vi "CRYSelect Signal Type Dialog.vi"(6 "Channel Info In":T1[](array[typedef]) {"Coupling" items=["Default"=-1, "RSE"=10083, "NRSE"=10078, "Differential"=10106, "Pseudodifferential"=12529]; "term config" items=["Default"=-1, "RSE"=10083, "NRSE"=10078, "Differential"=10106, "Pseudodifferential"=12529]; "Anti-aliasing Factor (%fs)" format="%.2f"}, 8 "Selected Signal Type In":string[](array[string]), 9 "Mode(0ne or More)":bool, 10 "I/O Calibration In":T5 {"Calibration 2D"."Sens Curve"."Z data" items=["dB", "Lin"]; "Calibration 2D"."Sens Curve"."X data" items=["dB", "Lin"]; "Calibration 2D"."Sens Curve"."Y data" items=["dB", "Lin"]; "Calibration 2D"."Sens Curve"."Z dB ref" format="%.1f"; "Calibration 2D"."Sens Curve"."Z axis" items=["Log", "Lin"]; "Calibration 2D"."Sens Curve"."X dB ref" format="%.1f"; "Calibration 2D"."Sens Curve"."X axis" items=["Log", "Lin"]; "Calibration 2D"."Sens Curve"."Y axis" items=["Log", "Lin"]; "Calibration 2D"."Sens Curve"."Y dB ref" format="%.1f"; "Calibration 2D"."Sens Curve"."Curve"."z" format="%.2f"; "Calibration 2D"."Sens Curve"."Curve"."y" format="%.2f"; "Calibration 2D"."Sens Curve"."Curve"."x" format="%.2f"; "Calibration 2D"."EQ Curve"."Z data" items=["dB", "Lin"]; "Calibration 2D"."EQ Curve"."X data" items=["dB", "Lin"]; "Calibration 2D"."EQ Curve"."Y data" items=["dB", "Lin"]; "Calibration 2D"."EQ Curve"."Z dB ref" format="%.1f"; "Calibration 2D"."EQ Curve"."Z axis" items=["Log", "Lin"]; "Calibration 2D"."EQ Curve"."X dB ref" format="%.1f"; "Calibration 2D"."EQ Curve"."X axis" items=["Log", "Lin"]; "Calibration 2D"."EQ Curve"."Y axis" items=["Log", "Lin"]; "Calibration 2D"."EQ Curve"."Y dB ref" format="%.1f"; "Calibration 2D"."EQ Curve"."Curve"."z" format="%.2f"; "Calibration 2D"."EQ Curve"."Curve"."y" format="%.2f"; "Calibration 2D"."EQ Curve"."Curve"."x" format="%.2f"; "Calibration 2D"."Corr Curve"."Z data" items=["dB", "Lin"]; "Calibration 2D"."Corr Curve"."X data" items=["dB", "Lin"]; "Calibration 2D"."Corr Curve"."Y data" items=["dB", "Lin"]; "Calibration 2D"."Corr Curve"."Z dB ref" format="%.1f"; "Calibration 2D"."Corr Curve"."Z axis" items=["Log", "Lin"]; "Calibration 2D"."Corr Curve"."X dB ref" format="%.1f"; "Calibration 2D"."Corr Curve"."X axis" items=["Log", "Lin"]; "Calibration 2D"."Corr Curve"."Y axis" items=["Log", "Lin"]; "Calibration 2D"."Corr Curve"."Y dB ref" format="%.1f"; "Calibration 2D"."Corr Curve"."Curve"."z" format="%.2f"; "Calibration 2D"."Corr Curve"."Curve"."y" format="%.2f"; "Calibration 2D"."Corr Curve"."Curve"."x" format="%.2f"; "Calibration 2D"."Calibration"."EQ Step size" items=["R10", "R20", "R40", "R80", "User"]; "Calibration 2D"."Calibration"."Corr Step size" items=["R10", "R20", "R40", "R80", "User"]}, 11 "In/Out Signal Type":bool) -> (1 "Calibration 2D Out":T2[](array[typedef]) {"Sens Curve"."Z data" items=["dB", "Lin"]; "Sens Curve"."X data" items=["dB", "Lin"]; "Sens Curve"."Y data" items=["dB", "Lin"]; "Sens Curve"."Z dB ref" format="%.1f"; "Sens Curve"."Z axis" items=["Log", "Lin"]; "Sens Curve"."X dB ref" format="%.1f"; "Sens Curve"."X axis" items=["Log", "Lin"]; "Sens Curve"."Y axis" items=["Log", "Lin"]; "Sens Curve"."Y dB ref" format="%.1f"; "Sens Curve"."Curve"."z" format="%.2f"; "Sens Curve"."Curve"."y" format="%.2f"; "Sens Curve"."Curve"."x" format="%.2f"; "EQ Curve"."Z data" items=["dB", "Lin"]; "EQ Curve"."X data" items=["dB", "Lin"]; "EQ Curve"."Y data" items=["dB", "Lin"]; "EQ Curve"."Z dB ref" format="%.1f"; "EQ Curve"."Z axis" items=["Log", "Lin"]; "EQ Curve"."X dB ref" format="%.1f"; "EQ Curve"."X axis" items=["Log", "Lin"]; "EQ Curve"."Y axis" items=["Log", "Lin"]; "EQ Curve"."Y dB ref" format="%.1f"; "EQ Curve"."Curve"."z" format="%.2f"; "EQ Curve"."Curve"."y" format="%.2f"; "EQ Curve"."Curve"."x" format="%.2f"; "Corr Curve"."Z data" items=["dB", "Lin"]; "Corr Curve"."X data" items=["dB", "Lin"]; "Corr Curve"."Y data" items=["dB", "Lin"]; "Corr Curve"."Z dB ref" format="%.1f"; "Corr Curve"."Z axis" items=["Log", "Lin"]; "Corr Curve"."X dB ref" format="%.1f"; "Corr Curve"."X axis" items=["Log", "Lin"]; "Corr Curve"."Y axis" items=["Log", "Lin"]; "Corr Curve"."Y dB ref" format="%.1f"; "Corr Curve"."Curve"."z" format="%.2f"; "Corr Curve"."Curve"."y" format="%.2f"; "Corr Curve"."Curve"."x" format="%.2f"; "Calibration"."EQ Step size" items=["R10", "R20", "R40", "R80", "User"]; "Calibration"."Corr Step size" items=["R10", "R20", "R40", "R80", "User"]}, 2 "Selected Signal Type":i32[](array[numeric]), 3 "Selected Flag":bool, 4 "Selected Channel Info Out":T1[](array[typedef]) caption="Selected I_channel Info" {"Coupling" items=["Default"=-1, "RSE"=10083, "NRSE"=10078, "Differential"=10106, "Pseudodifferential"=12529]; "term config" items=["Default"=-1, "RSE"=10083, "NRSE"=10078, "Differential"=10106, "Pseudodifferential"=12529]; "Anti-aliasing Factor (%fs)" format="%.2f"})   [LabVIEW 2013]
uses:
  Typedef Control/CRYCalibration All Cluster.ctl
  Typedef Control/CRYCalibration 2DCluster.ctl
  Typedef Control/CRYCalibration Cluster.ctl
  Typedef Control/CRYData Cluster.ctl
  Typedef Control/CRYHardware Channel Info.ctl
panel:
  in  "Select Signal Type(s)":i32[](listbox)
  in  "Cancel":bool
  in  "OK":bool
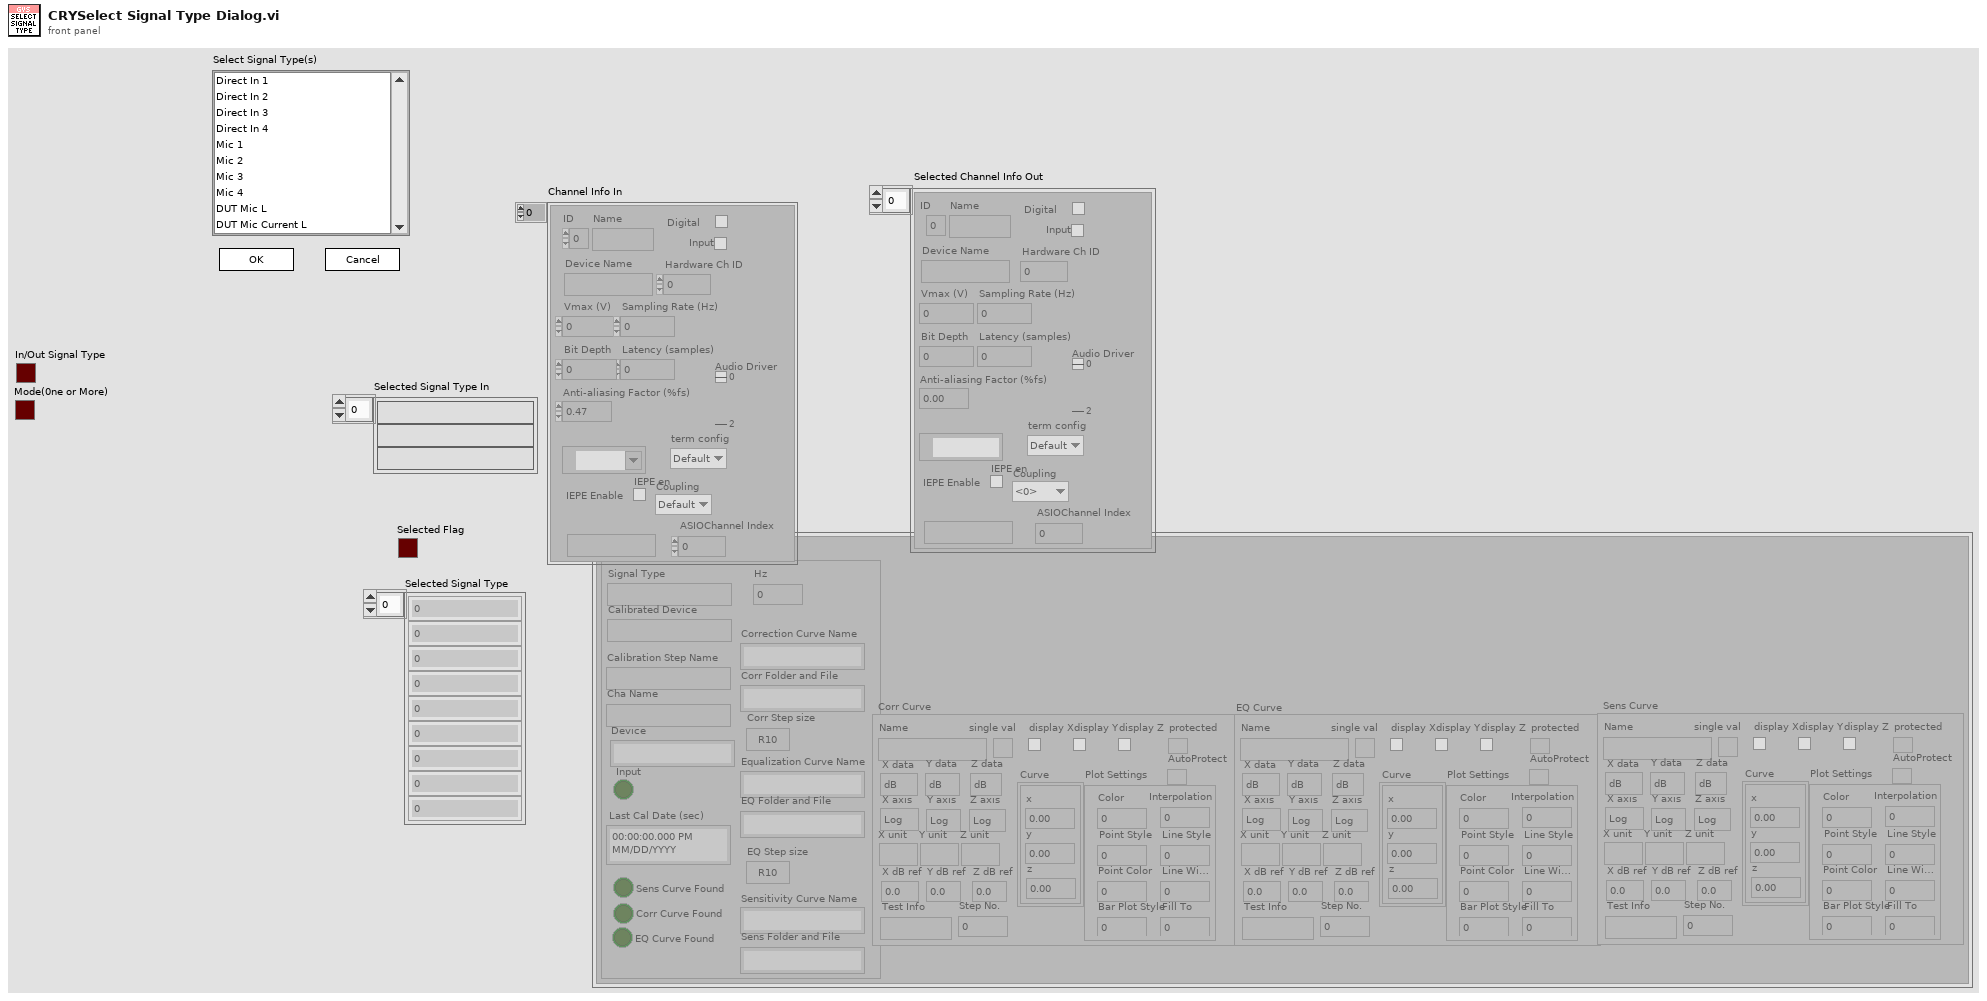
[diagram p1: front panel]
types:
  T1 = typedef "CRYHardware Channel Info.ctl" = cluster{"ID":i32, "Name":string, "Digital":bool, "Input":bool, "Device Name":string, "Hardware Ch ID":u8, "Vmax (V)":dbl, "Latency (samples)":dbl, "Sampling Rate (Hz)":u32, "Bit Depth":u32, "Anti-aliasing Factor (%fs)":sgl, "DAQmx Channel":tag, "term config":i32, "Coupling":i32, "IEPE en":bool, "ASIOChannel Name":string, "Audio Driver":u16, "ASIOChannel Index":u8}
  T2 = typedef "CRYCalibration 2DCluster.ctl" = cluster{"Calibration":T3, "Corr Curve":T4, "EQ Curve":T4, "Sens Curve":T4}
  T3 = typedef "CRYCalibration Cluster.ctl" = cluster{"Calibration Step Name":string, "Device":string, "Correction Curve Name":string, "Equalization Curve Name":string, "Sensitivity Curve Name":string, "Corr Folder and File":string, "EQ Folder and File":string, "Sens Folder and File":string, "Corr Step size":u16, "EQ Step size":u16, "Input":bool, "Last Cal Date (sec)":timestamp, "Cha Name":string, "Corr Curve Found":bool, "EQ Curve Found":bool, "Sens Curve Found":bool, "Signal Type":string, "Calibrated Device":string, "Hz":u32}
  T4 = typedef "CRYData Cluster.ctl" = cluster{"Name":string, "Curve":cluster{"x":dbl, "y":dbl, "z":dbl}[], "X data":u16, "Y data":u16, "Z data":u16, "X axis":u16, "Y axis":u16, "Z axis":u16, "X unit":string, "Y unit":string, "Z unit":string, "X dB ref":dbl, "Y dB ref":dbl, "Z dB ref":dbl, "single val":bool, "protected":bool, "display X":bool, "display Y":bool, "display Z":bool, "Test Info":string, "Step No.":i32, "Plot Settings":cluster{"Color":u32, "Interpolation":u8, "Point Style":u8, "Line Style":u8, "Point Color":u32, "Line Width":u8, "Bar Plot Style":u8, "Fill To":i16}, "AutoProtect":bool}
  T5 = typedef "CRYCalibration All Cluster.ctl" = cluster{"Calibration 2D":T2[], "Help":string, "Tab Value":i32, "Input Signal Type":string, "Output Signal Type":string}
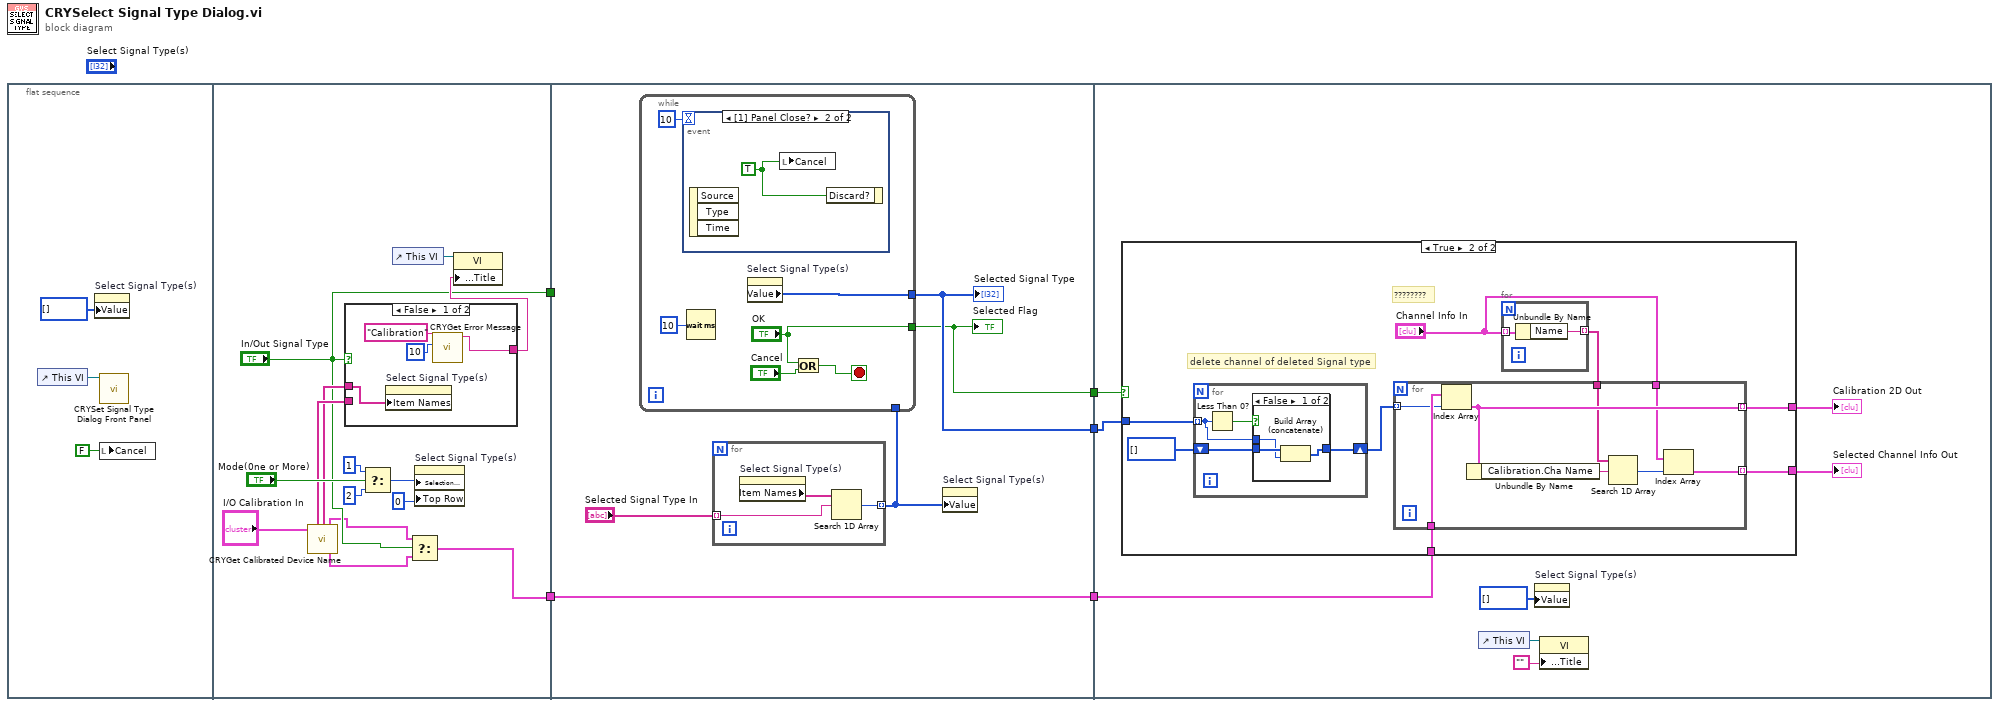
[diagram p0: block diagram]
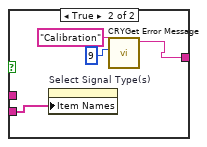
[diagram p2: hidden frame]
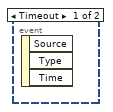
[diagram p3: hidden frame]
diagram:
  n1 = flat-sequence {
    tunnel: ["In/Out Signal Type"] -> w4
    tunnel: [w10] -> w3
    tunnel: [w35] -> w5
    tunnel: w4 -> [_]
    tunnel: w3 -> [w33]
    tunnel: [w33] -> w2
    tunnel: [w32] -> w1
    tunnel: w5 -> [w47]
    tunnel: w2 -> [w48]
    tunnel: w1 -> [w46]
    frame #0 {
      n2 = control-ref of="This VI"() -> (w7:refnum<vi>)
      n3 = property on="Select Signal Type(s)" class="LstBox (strict)"("Value"=i32[] [] ("Select channel(s)")) -> ()  [unwired: 2 in, 2 out]
      n4 = call "CRYSet Signal Type Dialog Front Panel.vi"("Vi Ref"=w7) -> ()  [unwired: 11 in]
      n5 = local write "Cancel"(FALSE ("Cancel")) -> ()
    }
    frame #1 {
      n6 = call "CRYGet Calibrated Device Name.vi"("Calibration"="I/O Calibration In") -> ("I_Signal Type Out"=w15:string[], "O_Signal Type Out"=w14:string[], "I_Calibration Out"=w12:T2[], "O_Calibration Out"=w11:T2[])  [unwired: 7 in, 4 out]
      n7 = case shown="False" "In/Out Signal Type" {
        tunnel: w14 -> [w23 _]
        tunnel: [w24 w28] -> w21
        tunnel: w15 -> [_ w27]
        frame False {
          n8 = property on="Select Signal Type(s)" class="LstBox (strict)"("Item Names"=w23) -> ()  [unwired: 2 in, 2 out]
          n9 = call "CRYGet Error Message.vi"("Error No"=10, "Kind"="Calibration") -> ("Message"=w24:string)  [unwired: 4 in, 5 out]
        }
        frame True {
          n10 = property on="Select Signal Type(s)" class="LstBox (strict)"("Item Names"=w27) -> ()  [unwired: 2 in, 2 out]
          n11 = call "CRYGet Error Message.vi"("Error No"=9, "Kind"="Calibration") -> ("Message"=w28:string)  [unwired: 4 in, 5 out]
        }
      }
      n12 = Select(t=1 ("Selection Mode"), s="Mode(0ne or More)", f=2 ("Selection Mode")) -> (s? t:f=w17:i32)
      n13 = control-ref of="This VI"() -> (w22:refnum<vi>)
      n14 = Select(t=w12, s="In/Out Signal Type", f=w11) -> (s? t:f=w10:T2[])
      n15 = property on="Select Signal Type(s)" class="LstBox (strict)"("Selection Mode"=w17, "Top Row"=0) -> ()  [unwired: 2 in, 2 out]
      n16 = property class="VI"(reference=w22, "Front Panel.Title"=w21) -> ()  [unwired: 1 in, 2 out]
    }
    frame #2 {
      n17 = for {
        tunnel: "Selected Signal Type In" -> [w37] mode=indexing
        tunnel: [w36] -> w31 mode=indexing
        n18 = property on="Select Signal Type(s)" class="LstBox (strict)"() -> ("Item Names"=w38:string[])  [unwired: 2 in, 2 out]
        n19 = Search 1D Array(1D array=w38, element=w37) -> (index of element=w36:i32)  [unwired: 1 out]
      }
      n20 = while {
        tunnel: ["OK"] -> w32
        tunnel: [w40] -> w35
        tunnel: w31 -> [_]
        stop <- w44 stop-if-true
        n21 = event shown="[1] Panel Close?" {
          selector: _ -> [_ _]
          dyn-events: _ -> [_ _]
          timeout: 10 -> [_ _]
          event Timeout {
            n22 = event-data() -> ()  [unwired: 1 in, 3 out]
          }
          event Panel Close? {
            w45 = TRUE ("OK")
            n23 = event-data() -> ()  [unwired: 1 in, 3 out]
            n24 = local write "Cancel"(w45) -> ()
            n25 = event-data("Discard?"=w45) -> ()  [unwired: 1 in, 1 out]
          }
        }
        n26 = Wait (ms)(milliseconds to wait=u32 10 ("millisecond multiple")) -> ()  [unwired: 1 out]
        n27 = property on="Select Signal Type(s)" class="LstBox (strict)"() -> ("Value"=w40:i32[])  [unwired: 2 in, 2 out]
        n28 = Or(x="OK", y="Cancel") -> (x .or. y?=w44:bool)
      }
      "Selected Flag" <- w32
      "Selected Signal Type" <- w35
      n29 = property on="Select Signal Type(s)" class="LstBox (strict)"("Value"=w31) -> ()  [unwired: 2 in, 2 out]
    }
    frame #3 {
      n30 = case shown="True" w46 {
        tunnel: [_ w61] -> w50
        tunnel: [_ w58] -> w49
        tunnel: w48 -> [_ w57]
        tunnel: w47 -> [_ w56]
        frame False {
        }
        frame True {
          # "delete channel of deleted Signal type"
          # "????????"
          n31 = for {
            tunnel: w56 -> [w62] mode=indexing
            shift-right: [w64] -> w54
            shift-left: i32[] [] ("Value") -> [w63]
            n32 = Less Than 0?(x=w62) -> (x < 0?=w65:bool)
            n33 = case shown="False" w65 {
              tunnel: [w66 w69] -> w64
              tunnel: w63 -> [w68 w69]
              tunnel: w62 -> [w67 _]
              frame False {
                n34 = Build Array (concatenate)(w68, w67) -> (w66:i32[])
              }
              frame True {
              }
            }
          }
          n35 = for {
            tunnel: "Channel Info In" -> [w71] mode=indexing
            tunnel: [w70] -> w60 mode=indexing
            n36 = Unbundle By Name(w71) -> ("Name"=w70:string)
          }
          n37 = for {
            tunnel: [w79] -> w61 mode=indexing
            tunnel: w60 -> [w78]
            tunnel: "Channel Info In" -> [w75]
            tunnel: [w74] -> w58 mode=indexing
            tunnel: w57 -> [w73]
            tunnel: w54 -> [w72] mode=indexing
            n38 = Index Array(array=w73, index=w72) -> (element=w79:T2)
            n39 = Unbundle By Name(w79) -> ("Calibration.Cha Name"=w77:string)
            n40 = Search 1D Array(1D array=w78, element=w77) -> (index of element=w76:i32)  [unwired: 1 in]
            n41 = Index Array(array=w75, index=w76) -> (element=w74:T1)
          }
        }
      }
      "Calibration 2D Out" <- w50
      "Selected Channel Info Out" <- w49
      n42 = control-ref of="This VI"() -> (w53:refnum<vi>)
      n43 = property on="Select Signal Type(s)" class="LstBox (strict)"("Value"=i32[] [] ("Select channel(s)")) -> ()  [unwired: 2 in, 2 out]
      n44 = property class="VI"(reference=w53, "Front Panel.Title"="") -> ()  [unwired: 1 in, 2 out]
    }
  }
